vi "Self Execution.vi"(4 "Any Data 2":variant, 6 "Any Data":variant, 8 "error in (no error)":errorcluster, 9 "Task Ancestor In":refnum<class "Task Ancestor.lvclass">, 10 "Message In":refnum<class "Message.lvclass">, 11 "Actor In":refnum<class "System Actor.lvclass">) -> (0 "error out":errorcluster, 1 "Task Ancestor Out":refnum<class "Task Ancestor.lvclass">, 2 "Message Out":refnum<class "Message.lvclass">, 3 "Actor Out":refnum<class "System Actor.lvclass">)   [LabVIEW 2024, in "Task Ancestor.lvclass"]
uses:
  Task Ancestor.lvclass
  Actor/System Actor/System Actor.lvclass
  Message/Message.lvclass
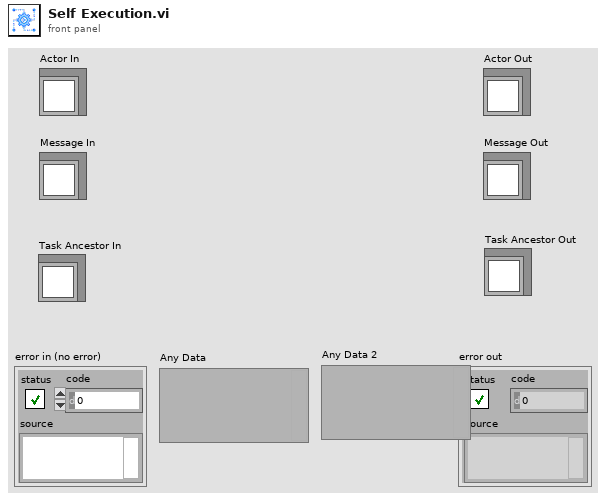
[diagram p1: front panel]
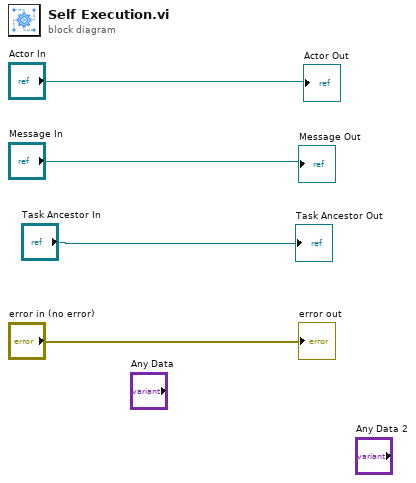
[diagram p0: block diagram]
diagram:
  "error out" <- "error in (no error)"
  "Message Out" <- "Message In"
  "Task Ancestor Out" <- "Task Ancestor In"
  "Actor Out" <- "Actor In"
